vi "Dashboard Main.vi"() -> ()   [LabVIEW 2017]
uses:
  <vilib>/Utility/miscctls.llb/LVRowAndColumnTypeDef.ctl
  <vilib>/event_ctls.llb/eventvkey.ctl
  <vilib>/MakerHub/LINX/Public/Peripherals/Digital/Digital Write 1 Chan.vi
  <vilib>/MakerHub/LINX/Public/Peripherals/Digital/Digital Write N Chans.vi
  <vilib>/MakerHub/LINX/Private/Local IO/LinxDigitalWrite.vi
  <vilib>/MakerHub/LINX/Public/Utilities/Check Channel.vi
  <vilib>/Rock Robotics/Network Tables/NT Read Numeric Array.vi
  <vilib>/Rock Robotics/WPI/Dashboard/WPI_DashboardLogging Global.vi
  <vilib>/MakerHub/LINX/Public/Utilities/Open Serial.vi
  <vilib>/Rock Robotics/Network Tables/NT Read Boolean.vi
  <vilib>/MakerHub/LINX/Private/Utilties/Generate Error.vi
  <vilib>/MakerHub/LINX/LMH-LINX.lvlib
panel:
  in  "Camera Settings Right":T1={"Frame Rate"=30, "Compression"=30, "Size"=1, "DB Camera Config"=FALSE} {"Frame Rate" scale=1.0..30.0; "Compression" scale=100.0..-1.0; "Size" items=["640x480", "320x240", "160x120"]}
  in  "Camera Name Right":string(combo)="No Camera Selection"
  out "Camera Info":cluster{"Mbps LED":bool, "Mbps":dbl, "fps":dbl} {"fps" format="%#.1g"; "Mbps" format="%#.1g"}
  in  "Camera Settings":T1={"Frame Rate"=30, "Compression"=30, "Size"=1, "DB Camera Config"=FALSE} {"Frame Rate" scale=1.0..30.0; "Compression" scale=100.0..-1.0; "Size" items=["640x480", "320x240", "160x120"]}
  in  "TCP":refnum<k5>
  in  "Rec Mode":enum32{"Stop", "Record", "Playback"}(radio)
  out "Robot IP":string
  out "Image Message":string="Timeout in Camera Communications"
  in  "Dashboard Tab":T2(tab)
  in  "Select Auto":string(combo)="Select Autonomous ..."
  out "NT Connection":bool
  out "MotorChart R":cluster{"Numeric":dbl, "Numeric":dbl}(graph)
  out "MotorChart L":cluster{"Numeric":dbl, "Numeric":dbl}(graph)
  out "MotorSliders R":cluster{"MotorSlide1":dbl, "MotorSlide2":dbl} {"MotorSlide2" scale=-1.0..1.0 scale format="%#_2e"; "MotorSlide1" scale=-1.0..1.0 scale format="%#_2e"}
  out "MotorSliders L":cluster{"MotorSlide1":dbl, "MotorSlide2":dbl} {"MotorSlide2" scale=-1.0..1.0 scale format="%#_2e"; "MotorSlide1" scale=-1.0..1.0 scale format="%#_2e"}
  out "Gyro":dbl(knob) scale=0.0..360.0
  out "JS1 Z":dbl(slide) scale=-1.0..1.0 scale format="%#_2e"
  out "JS1 Graph":cluster{"X":dbl, "Y":dbl}[](graph)
  out "JS1 Buttons":T3
  out "JS2 Z":dbl(slide) scale=-1.0..1.0 scale format="%#_2e"
  out "JS2 Graph":cluster{"X":dbl, "Y":dbl}[](graph)
  out "JS2 Buttons":T3
  out "Mode":T4(ring)=enum."Auto Disabled"
  out "Camera Image Right":T5(plugin-control)
  in  "DB/String 9":string
  in  "DB/String 8":string
  in  "DB/String 7":string
  in  "DB/String 6":string
  in  "DB/String 5":string
  in  "DB/String 4":string
  in  "DB/String 3":string
  in  "DB/String 2":string
  in  "DB/String 1":string
  in  "DB/String 0":string
  in  "DB/Slider 0":dbl(slide) scale=0.0..5.0
  in  "DB/Slider 1":dbl(slide) scale=0.0..5.0
  in  "DB/Slider 2":dbl(slide) scale=0.0..5.0
  in  "DB/Slider 3":dbl(slide) scale=0.0..5.0
  out "DB/LED 3":bool
  out "DB/LED 2":bool
  out "DB/LED 1":bool
  out "DB/LED 0":bool
  in  "DB/Button 3":bool
  in  "DB/Button 2":bool
  in  "DB/Button 1":bool
  in  "DB/Button 0":bool caption="New Name"
  in  "Test Slider":dbl(slide) scale=0.0..100.0 scale format="%#_3g"
  in  "On/Off":bool caption="Solenoid"
  in  "Test Name":u16(ring) items=["Select the test to run..."]
  in  "Test Tree":string(tree)
  in  "Motor":cluster{"Value":dbl, "Enable":bool} {"Value" scale=-1.0..1.0 scale format="%#_3g"}
  out "Progress":T6 {"Test Progress" scale=0.0..100.0}
  in  "Rev/Fwd":cluster{"Forward":bool, "Reverse":bool}
  in  "Test Ring":u16(ring) items=["Monochrome", "Color"]
  out "Cmd Status":string
  in  "Execute Command":bool
  in  "Command Params":string[][](table)
  in  "Command Selection":i32(listbox)
  in  "CheckList":i32(listbox)
  out "Tree":string(tree)
  out "Camera Image":T5(plugin-control)
  out "Background":bool
  in  "Camera Name":string(combo)="No Camera Selection"
  # "HW"
  # "HW"
  # "Joysticks"
  # "Drive Motors"
  # "Front"
  # "Right"
  # "Left"
  # "Back"
  # "This tab is a great place for autonomous settings and robot-specific values.\nPlace controls and indicators inside this tab and match name to\nDashboard Variables on robot. You can also delete this comment."
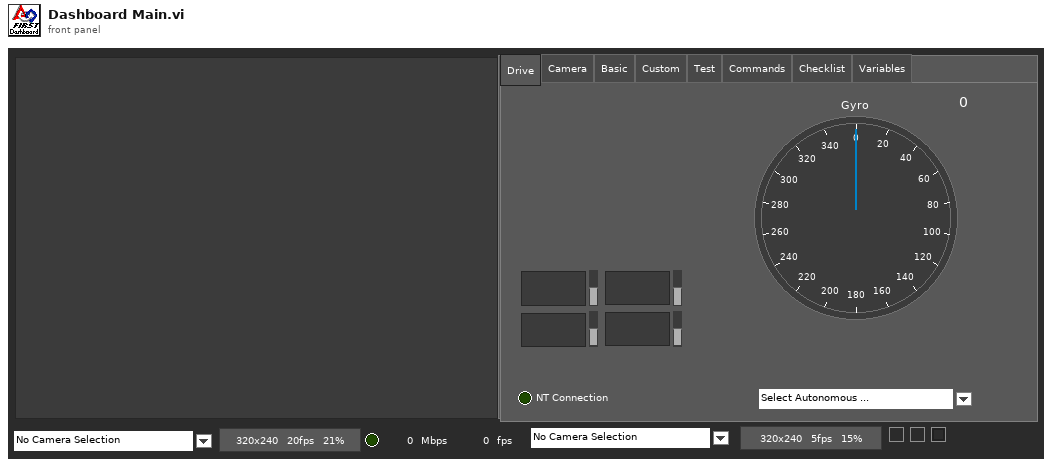
[diagram p1: front panel]
types:
  T1 = cluster{"Frame Rate":i32, "Compression":i32, "Size":u16, "DB Camera Config":bool}
  T2 = enum32{"Drive", "Camera", "Basic", "Custom", "Test", "Commands", "Checklist", "Variables"}
  T3 = cluster{bool, bool, bool, bool, bool, bool, bool, bool, bool, bool, bool, bool}
  T4 = enum8{"Tele-Op Disabled", "Tele-Op Enabled", "Auto Disabled", "Auto Enabled", "Test Disabled", "Test Enabled", "Disconnected", "No Code", "E-Stop"}
  T5 = typedef "IMAQ Image.ctl" = refnum<image>
  T6 = cluster{"Test Progress":u8, "Test Progress Text":string}
  T7 = cluster{"Save Path":path, "Interval (s)":dbl, "Keep":i32}
  T8 = typedef "Image Type" = u32
  T9 = cluster{"IDs":cluster{"RPC field ID":u16, "Unique ID":u16}, "String":string}
  T10 = typedef "LMH-LINX.lvlib/LINX Ref.ctl" = cluster{"IO":T11, "Interface":T12, "LINX Device Config":T13}
  T11 = typedef "LMH-LINX.lvlib/Platform.ctl" = enum16{"Remote", "Local"}
  T12 = typedef "LMH-LINX.lvlib/Interface.ctl" = enum16{"Serial", "TCP"}
  T13 = typedef "LMH-LINX.lvlib/Device.lvlib/LINX Device Config.ctl" = cluster{"Interface":T12, "COM Port":refnum<visa-resource-name>, "TCP Configuration":T14, "Device Family":u8, "Device ID":u8, "Device Name":string, "TCP Ref":refnum<k5>, "Channels":T15}
  T14 = typedef "LMH-LINX.lvlib/Device.lvlib/TCP Config.ctl" = cluster{"IP Address":string, "Port":u16}
  T15 = typedef "LMH-LINX.lvlib/Channels.ctl" = cluster{"DI":u8[], "DO":u8[], "AI":u8[], "AO":u8[], "PWM":u8[], "QE":u8[], "UART":u8[], "I2C 2":u8[], "SPI":u8[], "CAN":u8[], "Servo":u8[], "AI Ref (V)":dbl, "AI Resolution (Bits)":u8, "AO Ref (V)":dbl, "AO Resolution (Bits)":u8}
  T16 = cluster{"Error Strings":string, "Disable Counts":cluster{u16, u16}, "Rail Faults":cluster{u16, u16, u16}, "Robot IP":string, "DB Mode":u8, "Event Info":cluster{"Name":string, "Type":u8, "Number":u16, "Replay":u8}}
  T17 = cluster{"Storage":cluster{"Disk Free":u64, "RAM Block":u32, "RAM free":u32}, "CPU Utilization":cluster{"CPU % ISR":sgl, "CPU % Time Crit":sgl, "CPU % Timed Str":sgl, "CPU % High":sgl, "CPU % Above":sgl, "CPU % Normal":sgl, "CPU % Low":sgl}, "CAN":cluster{"% Bus Utilization":sgl, "Bus Off Cnt":u32, "TX_FIFO Full Cnt":u32, "Receive Error Cnt":u8, "Transmit Error Cnt":u8}, "HID":cluster{"HID Outputs":u32, "Rumble Low":u16, "Rumble High":u16}[]}
  T18 = cluster{"Status bits":cluster{"Test Mode":bool, "Autonomous":bool, "Enabled":bool, "Code Start":bool, "Brownout":bool, "Reserved 2":bool, "Reserved 3":bool, "E-Stop":bool}, "Code Trace":cluster{"Disabled":bool, "TeleOp":bool, "Auto":bool, "Test":bool}, "Controller Type":enum16{"unknown", "cRIO", "roboRio"}, "Code?":enum16{"unknown", "noCode", "code"}, "Battery V":dbl}
  T19 = cluster{"Control Bits":cluster{"TestMode":bool, "Autonomous":bool, "Enabled":bool, "FMS Present":bool, bool, bool, bool, "E-Stop":bool}, "Team Station ":u8, "Countdown":sgl, "Joystick Values":cluster{"Axes":dbl[], "Buttons":bool[], "POVs":i16[]}[]}
  T20 = cluster{"Axes":dbl[], "Buttons":bool[], "POVs":i16[]}[]
  T21 = cluster{"Axes":dbl[], "Buttons":bool[], "POVs":i16[]}
  T22 = cluster{"Buttons[0]":bool, "Buttons[1]":bool, "Buttons[2]":bool, "Buttons[3]":bool, "Buttons[4]":bool, "Buttons[5]":bool, "Buttons[6]":bool, "Buttons[7]":bool, "Buttons[8]":bool, "Buttons[9]":bool, "Buttons[10]":bool, "Buttons[11]":bool}
  T23 = cluster{"Camera Image":refnum<vi>, "Dashboard Tab":refnum<vi>, "Background":refnum<vi>, "Rec Mode":refnum<vi>, "Test Slider":refnum<vi>, "On/Off ":refnum<vi>, "Test Ring":refnum<vi>, "Rev/Fwd":refnum<vi>, "Test Name":refnum<vi>, "Motor":refnum<vi>, "Progress":refnum<vi>, "CheckList":refnum<vi>, "Tree":refnum<vi>, "Test Tree":refnum<vi>, "Command Params":refnum<vi>, "Command Selection":refnum<vi>, "Execute Command":refnum<vi>, "Cmd Status":refnum<vi>, "Camera Settings":refnum<vi>, "Camera Name":refnum<vi>, "Camera Info":refnum<vi>, "Camera Settings Right":refnum<vi>, "Camera Name Right":refnum<vi>, "Camera Image Right":refnum<vi>}
  T24 = cluster{"Camera Name":string, string, "Saved DB Images Info":cluster{"Save Path":path, "Interval (s)":dbl, "Keep":i32}}
  T25 = cluster{"Camera Name Right":string, string, "Saved DB Images Info":cluster{"Save Path":path, "Interval (s)":dbl, "Keep":i32}}
  T26 = cluster{"Operation":enum16{"Update", "Clear"}, "Color Box":u32}[]
  T27 = typedef "eventvkey.ctl" = enum16{"ASCII", "Enter", "Return", "Shift", "Ctrl", "Alt", "Cmd", "Opt", "Caps", "NumLock", "Clear", "Break", "Up", "Down", "Left", "Right", "Insert", "Delete", "Home", "End", "PageUp", "PageDown", "Escape", "Help", "Pause", "ScrollLock", "F1", "F2", "F3", "F4", "F5", "F6", "F7", "F8", "F9", "F10", "F11", "F12", "F13", "F14", "F15", "F16", "F17", "F18", "F19", "F20", "F21", "F22", "F23", "F24", "Play", "VolumeUp", "VolumeDown", "Mute", "Two Byte Char"}
  T28 = cluster{"Image Size":bool, "Image Type":bool, "Pixel Value":bool, "ROI Information":bool, "Zoom Factor":bool}
  T29 = cluster{"Operation":enum16{"Update", "Clear"}, "Color Box":u32}
  T30 = typedef "LVRowAndColumnTypeDef.ctl" = cluster{"Row":i32, "Column":i32}
  T31 = cluster{"Shift":bool, "Ctrl":bool, "Alt":bool, "Cmd":bool, "Opt":bool}
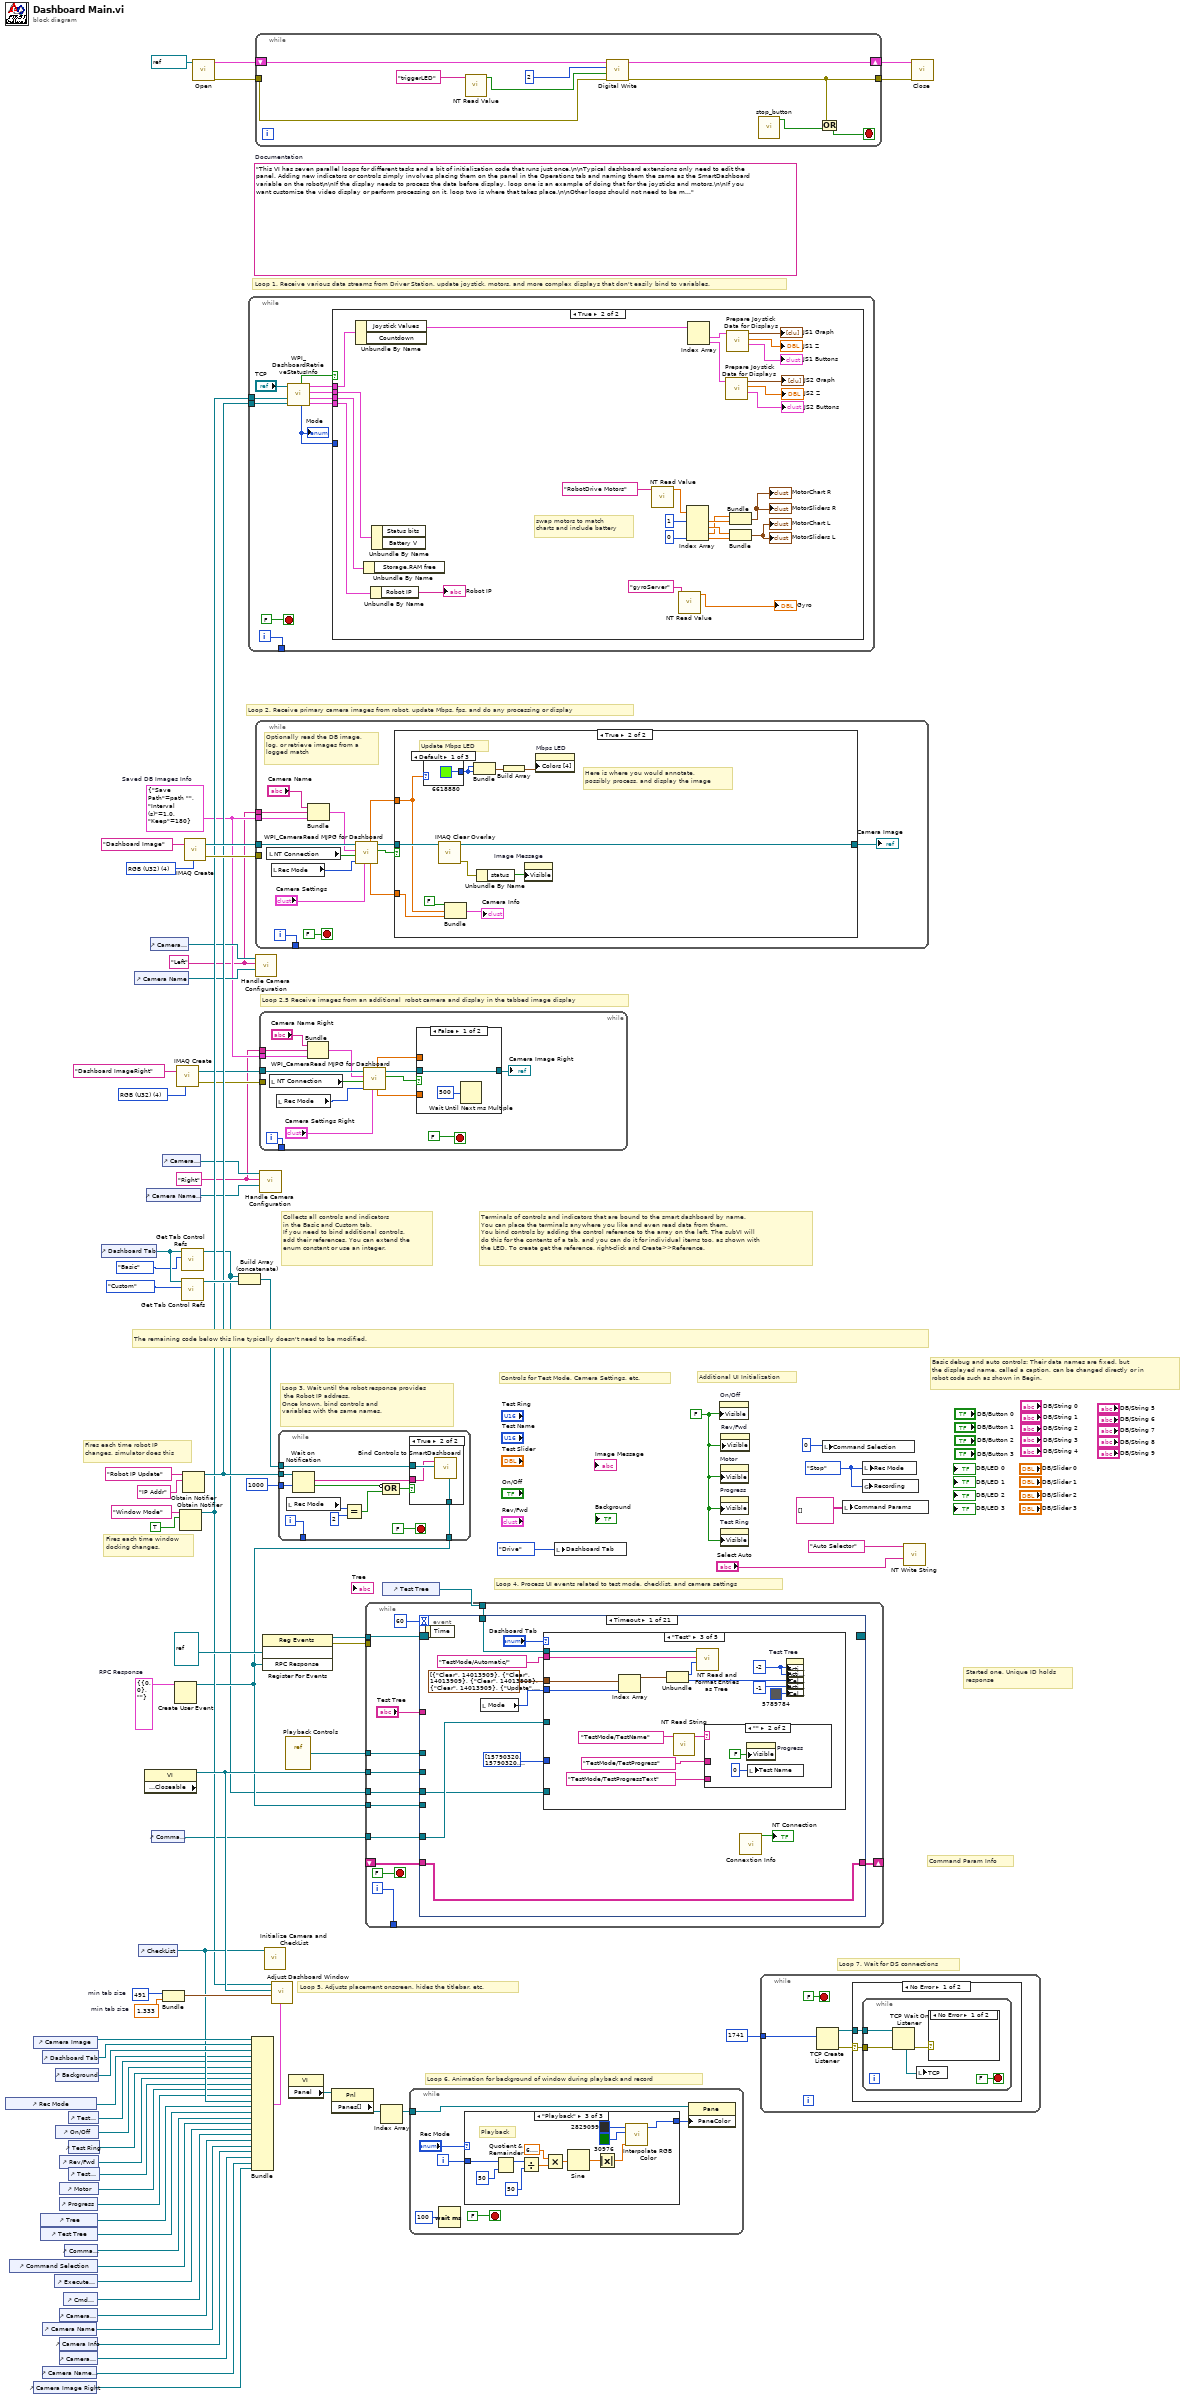
[diagram p0: block diagram]
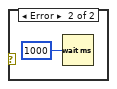
[diagram p3: hidden frame]
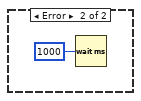
[diagram p4: hidden frame]
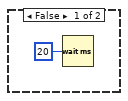
[diagram p5: hidden frame]
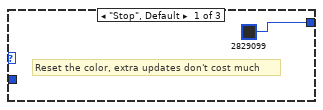
[diagram p6: hidden frame]
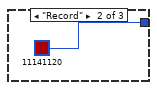
[diagram p7: hidden frame]
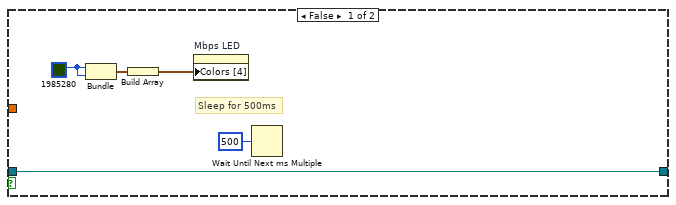
[diagram p9: hidden frame]
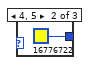
[diagram p10: hidden frame]
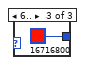
[diagram p11: hidden frame]
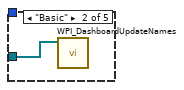
[diagram p13: hidden frame]
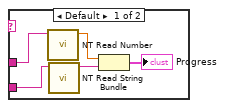
[diagram p14: hidden frame]
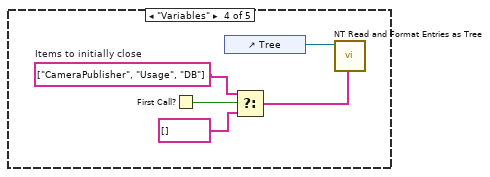
[diagram p15: hidden frame]
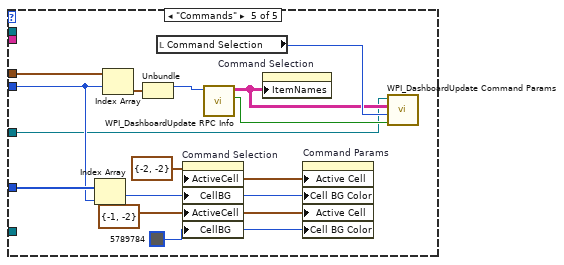
[diagram p16: hidden frame]
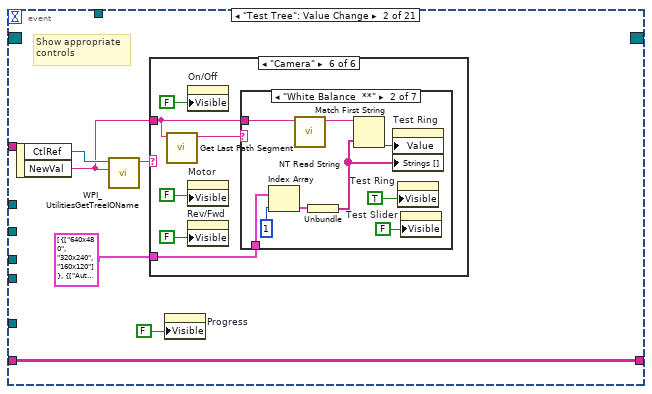
[diagram p17: hidden frame]
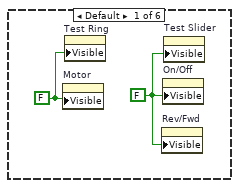
[diagram p18: hidden frame]
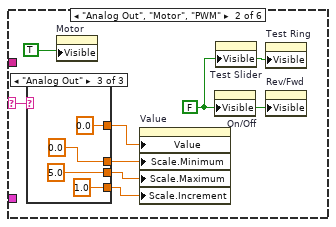
[diagram p19: hidden frame]
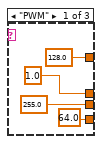
[diagram p20: hidden frame]
diagram:
  w8 = T7 {"Save Path"=path "", "Interval (s)"=1.0, "Keep"=180}  # Saved DB Images Info
  w7 = "Right"
  w6 = "Left"
  w18 = T8 4 items=["Grayscale (U8)", "Grayscale (I16)", "Grayscale (SGL)", "Complex (CSG)", "RGB (U32)", "HSL (U32)", "RGB (U64)"] ("Image Type")
  w34 = T9 {"IDs"={"RPC field ID"=0, "Unique ID"=0}, "String"=""}  # RPC Response
  w57 = 491  # min tab size
  w56 = 1.333  # min tab size
  w64 = enum32{"Stop", "Record", "Playback"}."Stop" ("Rec Mode")
  w41 = FALSE ("Visible")
  (unwired) "This VI has seven parallel loops for different tasks and a bit of initialization code that runs just once.\n\nTypical dashboard extensions only need to edit the panel. Adding new indicators or controls simply involves placing them on the panel in the Operations tab and naming them the same as the SmartDashboard variable on the robot\n\nIf the display needs to process the data before display, loop one is an example of doing that for the joysticks and motors.\n\nIf you want customize the video display or perform processing on it, loop two is where that takes place.\n\nOther loops should not need to be modified. They are pretty standard, and document the task they perform."  # Documentation
  w81 = T8 4 items=["Grayscale (U8)", "Grayscale (I16)", "Grayscale (SGL)", "Complex (CSG)", "RGB (U32)", "HSL (U32)", "RGB (U64)"] ("Image Type")
  # "Loop 2.5 Receive images from an additional  robot camera and display in the tabbed image display"
  # "Command Param Info"
  # "Started one, Unique ID holds\nresponse"
  # "Loop 7. Wait for DS connections"
  # "Basic debug and auto controls: Their data names are fixed, but\nthe displayed name, called a caption, can be changed directly or in\nrobot code such as shown in Begin."
  # "Controls for Test Mode, Camera Settings, etc."
  # "Additional UI Initialization"
  # "Loop 6. Animation for background of window during playback and record"
  # "Fires each time robot IP\nchanges, simulator does this"
  # "Fires each time window\ndocking changes."
  # "Collects all controls and indicators\nin the Basic and Custom tab.\nIf you need to bind additional controls,\nadd their references. You can extend the\nenum constant or use an integer."
  # "The remaining code below this line typically doesn't need to be modified."
  # "Loop 4. Process UI events related to test mode, checklist, and camera settings"
  # "Terminals of controls and indicators that are bound to the smart dashboard by name.\nYou can place the terminals anywhere you like and even read data from them.\nYou bind controls by adding the control reference to the array on the left. The subVI will\ndo this for the contents of a tab, and you can do it for individual items too, as shown with\nthe LED. To create get the reference, right-click and Create>>Reference."
  # "Loop 3. Wait until the robot response provides\n the Robot IP address.\nOnce known, bind controls and\nvariables with the same names."
  # "Loop 5. Adjusts placement onscreen, hides the titlebar, etc."
  # "Loop 1. Receive various data streams from Driver Station, update joystick, motors, and more complex displays that don't easily bind to variables."
  # "Loop 2. Receive primary camera images from robot, update Mbps, fps, and do any processing or display"
  n1 = control-ref of="Rec Mode"() -> (w47:refnum<vi>)
  n2 = control-ref of="Command Selection"() -> (w33:refnum<vi>)
  n3 = control-ref of="Camera Image Right"() -> (w11:refnum<vi>)
  n4 = control-ref of="Camera Image"() -> (w59:refnum<vi>)
  n5 = control-ref of="Tree"() -> (w51:refnum<vi>)
  n6 = control-ref of="Test Tree"() -> (w50:refnum<vi>)
  n7 = control-ref of="Dashboard Tab"() -> (w58:refnum<vi>)
  n8 = control-ref of="Camera Name"() -> (w24:refnum<vi>)
  n9 = control-ref of="Camera Name Right"() -> (w12:refnum<vi>)
  n10 = control-ref of="Execute Command"() -> (w35:refnum<vi>)
  n11 = control-ref of="Background"() -> (w54:refnum<vi>)
  n12 = control-ref of="On/Off"() -> (w45:refnum<vi>)
  n13 = control-ref of="Progress"() -> (w42:refnum<vi>)
  n14 = control-ref of="Camera Settings"() -> (w25:refnum<vi>)
  n15 = control-ref of="Camera Info"() -> (w23:refnum<vi>)
  n16 = control-ref of="Camera Settings Right"() -> (w13:refnum<vi>)
  n17 = control-ref of="Rev/Fwd"() -> (w43:refnum<vi>)
  n18 = control-ref of="Motor"() -> (w48:refnum<vi>)
  n19 = control-ref of="Cmd Status"() -> (w29:refnum<vi>)
  n20 = control-ref of="Command Params"() -> (w36:refnum<vi>)
  n21 = control-ref of="Test Slider"() -> (w46:refnum<vi>)
  n22 = control-ref of="Test Ring"() -> (w44:refnum<vi>)
  n23 = control-ref of="Test Name"() -> (w49:refnum<vi>)
  n24 = control-ref of="Dashboard Tab"() -> (w62:refnum<vi>)
  n25 = control-ref of="Camera Name"() -> (w26:refnum<vi>)
  n26 = control-ref of="CheckList"() -> (w52:refnum<vi>)
  n27 = property class="VI" props=["Front Panel.Closeable"]() -> (reference out=w63:refnum<vi>)  [unwired: 2 in, 2 out]
  n28 = control-ref of="Camera Name Right"() -> (w14:refnum<vi>)
  n29 = control-ref of="Camera Settings"() -> (w27:refnum<vi>)
  n30 = control-ref of="Command Params"() -> (w28:refnum<vi>)
  n31 = control-ref of="Camera Settings Right"() -> (w15:refnum<vi>)
  n32 = Bundle("min tab size"=w57, "min tab size"=w56) -> (w55:cluster{"min tab size":i32, "min tab size":dbl})  [unwired: 1 in]
  n33 = Create User Event(user event datatype=w34) -> (user event=w30:refnum<user-event>)  [unwired: 1 in, 1 out]
  n34 = call "IMAQ Create"("Image Name"="Dashboard ImageRight", "Image Type"=w18) -> ("New Image"=w17:T5, "error out"=w16:errorcluster)  [unwired: 2 in, 1 out]
  n35 = Obtain Notifier(name (unnamed)="Window Mode", notification data type=TRUE) -> (notifier out=w39:refnum<notifier>)  [unwired: 2 in, 2 out]
  n36 = call <vilib>:"Get Tab Control Refs.vi"("Page Index"=T2."Basic" ("Dashboard Tab"), "TabControl in"=w62) -> ("ControlsOnPage"=w22:refnum<vi>[])  [unwired: 9 in]
  n37 = call <vilib>:"Get Tab Control Refs.vi"("Page Index"=T2."Custom" ("Dashboard Tab"), "TabControl in"=w62) -> ("ControlsOnPage"=w61:refnum<vi>[])  [unwired: 9 in]
  n38 = Obtain Notifier(name (unnamed)="Robot IP Update", notification data type="IP Addr" ("name (unnamed)")) -> (notifier out=w40:refnum<notifier>)  [unwired: 2 in, 2 out]
  n39 = call "IMAQ Create"("Image Name"="Dashboard Image", "Image Type"=w81) -> ("New Image"=w79:T5, "error out"=w78:errorcluster)  [unwired: 2 in, 1 out]
  n40 = call-poly <vilib>:"Open.vi"("Serial Port"=refnum<visa-resource-name> "N/A") -> ("Error Out"=w3:errorcluster, "LINX Resource"=w4:T10)  [unwired: 8 in, 1 out]
  n41 = Build Array (concatenate)(w22, w61) -> (w60:refnum<vi>[])
  n42 = while {
    tunnel: [w91] -> _
    tunnel: w40 -> [w85]
    tunnel: w39 -> [w82]
    i -> [w91]
    stop <- FALSE stop-if-true
    n43 = call <vilib>:"WPI_DashboardRetrieveStatusInfo.vi"("Binding Refnum"=w85, "Window Mode Notifier"=w82, "TCP Cnx"="TCP") -> ("Power and Errors"=w86:T16, "Robot Metrics"=w89:T17, "Status Info"=w90:T18, "Control Info"=w87:T19, "Robot Mode"=w84:T4, "Process?"=w88:bool)  [unwired: 3 in]
    "Mode" <- w84
    n44 = case shown="True" w88 {
      tunnel: w90 -> [_ w119]
      tunnel: w89 -> [_ w118]
      tunnel: w87 -> [_ w117]
      tunnel: w86 -> [_ w116]
      tunnel: w84 -> [_ _]
      frame False {
        n45 = Wait (ms)(milliseconds to wait=u32 20) -> ()  [unwired: 1 out]
      }
      frame True {
        # "swap motors to match\ncharts and include battery"
        n46 = Unbundle By Name(w117) -> ("Joystick Values"=w107:T20)  [unwired: 1 out]
        n47 = Unbundle By Name(w118) -> ()  [unwired: 1 out]
        n48 = Unbundle By Name(w116) -> ("Robot IP"=→"Robot IP":string)
        n49 = Unbundle By Name(w119) -> ()  [unwired: 2 out]
        n50 = call-poly <vilib>:"NT Read Value.vi"("Name"="RobotDrive Motors") -> ("Numeric Array"=w97:dbl[])  [unwired: 9 in, 1 out]
        n51 = call-poly <vilib>:"NT Read Value.vi"("Name"="gyroServer") -> ("Numeric"=→"Gyro":dbl)  [unwired: 9 in, 1 out]
        n52 = Index Array(array=w97, index #1=1, index #4=0) -> (element #1=w111:dbl, element #2=w112:dbl, element #3=w110:dbl, element #4=w115:dbl)  [unwired: 2 in]
        n53 = Index Array(array=w107) -> (element #1=w106:T21, element #2=w102:T21)  [unwired: 2 in]
        n54 = call "Prepare Joystick Data for Displays.vi"("Joystick Values"=w102) -> ("Buttons"=→"JS2 Buttons":T22, "Z Axis"=→"JS2 Z":dbl, "Cartesian Data"=→"JS2 Graph":cluster{"X axis":dbl, "X axis":dbl}[])  [unwired: 8 in]
        n55 = call "Prepare Joystick Data for Displays.vi"("Joystick Values"=w106) -> ("Buttons"=→"JS1 Buttons":T22, "Z Axis"=→"JS1 Z":dbl, "Cartesian Data"=→"JS1 Graph":cluster{"X axis":dbl, "X axis":dbl}[])  [unwired: 8 in]
        n56 = Bundle("Numeric"=w110, "Numeric"=w111) -> (→"MotorChart R" →"MotorSliders R":cluster{"Numeric":dbl, "Numeric":dbl})  [unwired: 1 in]
        n57 = Bundle("Numeric"=w112, "Numeric"=w115) -> (→"MotorChart L" →"MotorSliders L":cluster{"Numeric":dbl, "Numeric":dbl})  [unwired: 1 in]
      }
    }
  }
  n58 = Bundle("Camera Image"=w59, "Dashboard Tab"=w58, "Background"=w54, "Rec Mode"=w47, "Test Slider"=w46, "On/Off"=w45, "Test Ring"=w44, "Rev/Fwd"=w43, "Test Name"=w49, "Motor"=w48, "Progress"=w42, "CheckList"=w52, "Tree"=w51, "Test Tree"=w50, "Command Params"=w36, "Command Selection"=w33, "Execute Command"=w35, "Cmd Status"=w29, "Camera Settings"=w25, "Camera Name"=w24, "Camera Info"=w23, "Camera Settings Right"=w13, "Camera Name Right"=w12, "Camera Image Right"=w11) -> (w53:T23)  [unwired: 1 in]
  n59 = call "Handle Camera Configuration.vi"("CameraNameRef"=w26, "Display Name"=w6, "ClusterRef"=w27) -> ()  [unwired: 9 in]
  n60 = while {
    shift-right: [w127] -> w2
    shift-left: w4 -> [w128]
    tunnel: w3 -> [w125]
    tunnel: [w126] -> w1
    stop <- w123 stop-if-true
    n61 = call-poly <vilib>:"NT Read Value.vi"("Name"="triggerLED") -> ("Boolean"=w120:bool)  [unwired: 9 in, 1 out]
    n62 = call-poly <vilib>:"Digital Write.vi"("Error In"=w125, "Output Value"=w120, "DO Channel"=u8 2 ("AO Channel"), "LINX Resource"=w128) -> ("Error Out"=w126:errorcluster, "LINX Resource"=w127:T10)  [unwired: 6 in]
    n63 = call "stop_button.vi"() -> ("Boolean"=w122:bool)  [unwired: 11 in]
    n64 = Or(x=w126, y=w122) -> (x .or. y?=w123:bool)
  }
  n65 = while {
    tunnel: w79 -> [w141]
    tunnel: w78 -> [_]
    tunnel: [w142] -> _
    tunnel: w8 -> [w132]
    tunnel: w6 -> [w129]
    i -> [w142]
    stop <- FALSE stop-if-true
    # "Optionally read the DB image,\nlog, or retrieve images from a\nlogged match"
    n66 = local read "NT Connection"() -> (w133:bool)
    n67 = local read "Rec Mode"() -> (w137:enum32{"Stop", "Record", "Playback"})
    n68 = Bundle("Camera Name"="Camera Name", w129, "Saved DB Images Info"=w132) -> (w131:T24)  [unwired: 1 in]
    n69 = call <vilib>:"WPI_CameraRead MJPG for Dashboard.vi"("Camera Settings"="Camera Settings", "Rec Mode"=w137, "NT Connection"=w133, "Capture Info"=w131, "Refnum in"=w141) -> ("Active"=w139:bool, "Refnum out"=w140:T5, "FPS"=w138:dbl, "Bandwidth (Mbps)"=w136:dbl)  [unwired: 3 in]
    n70 = case shown="True" w139 {
      tunnel: w140 -> [w144 w155]
      tunnel: w136 -> [_ w152]
      tunnel: w138 -> [_ w153]
      tunnel: [w144 w149] -> w134
      frame False {
        w146 = u32 1985280 ("Color Box")
        # "Sleep for 500ms"
        n71 = Bundle("Color Box"=w146, "Color Box"=w146) -> (w147:cluster{"Color Box":u32, "Color Box":u32})  [unwired: 1 out]
        n72 = Build Array(w147) -> (w145:cluster{"Color Box":u32, "Color Box":u32}[])
        n73 = property on="Mbps LED" class="Bool (strict)"("Colors [4]"=w145) -> ()  [unwired: 2 in, 2 out]
        n74 = Wait Until Next ms Multiple(millisecond multiple=u32 500) -> ()  [unwired: 1 out]
      }
      frame True {
        # "Here is where you would annotate,\npossibly process, and display the image"
        # "Update Mbps LED"
        n75 = case shown="Default" w152 {
          tunnel: [u32 6618880 ("Color Box") u32 16776722 ("Color Box") u32 16716800 ("Color Box")] -> w156
          frame Default {
          }
          frame 4, 5 {
          }
          frame 6.. {
          }
        }
        n76 = call "IMAQ Clear Overlay"("Image"=w155) -> ("error out"=w158:errorcluster, "Image Out"=w149:T5)  [unwired: 2 in, 7 out]
        n77 = Bundle(FALSE, "Bandwidth (Mbps)"=w152, "FPS"=w153) -> (→"Camera Info":cluster{bool, "Bandwidth (Mbps)":dbl, "FPS":dbl})  [unwired: 1 in]
        n78 = Bundle("Color Box"=w156, "Color Box"=w156) -> (w157:cluster{"Color Box":u32, "Color Box":u32})  [unwired: 1 out]
        n79 = Unbundle By Name(w158) -> ("status"=w159:bool)
        n80 = Build Array(w157) -> (w154:cluster{"Color Box":u32, "Color Box":u32}[])
        n81 = property on="Image Message" class="Str"("Visible"=w159) -> ()  [unwired: 2 in, 2 out]
        n82 = property on="Mbps LED" class="Bool (strict)"("Colors [4]"=w154) -> ()  [unwired: 2 in, 2 out]
      }
    }
    "Camera Image" <- w134
  }
  n83 = call "Handle Camera Configuration.vi"("CameraNameRef"=w14, "Display Name"=w7, "ClusterRef"=w15) -> ()  [unwired: 9 in]
  n84 = while {
    tunnel: w17 -> [w177]
    tunnel: w16 -> [_]
    tunnel: [w172] -> _
    tunnel: w8 -> [w166]
    tunnel: w7 -> [w163]
    i -> [w172]
    stop <- FALSE stop-if-true
    n85 = local read "NT Connection"() -> (w167:bool)
    n86 = local read "Rec Mode"() -> (w176:enum32{"Stop", "Record", "Playback"})
    n87 = Bundle("Camera Name Right"="Camera Name Right", w163, "Saved DB Images Info"=w166) -> (w165:T25)  [unwired: 1 in]
    n88 = call <vilib>:"WPI_CameraRead MJPG for Dashboard.vi"("Camera Settings"="Camera Settings Right", "Rec Mode"=w176, "NT Connection"=w167, "Capture Info"=w165, "Refnum in"=w177) -> ("Active"=w171:bool, "Refnum out"=w174:T5, "FPS"=w169:dbl, "Bandwidth (Mbps)"=w170:dbl)  [unwired: 3 in]
    n89 = case shown="False" w171 {
      tunnel: w174 -> [w178 w180]
      tunnel: w170 -> [_ _]
      tunnel: w169 -> [_ _]
      tunnel: [w178 w180] -> w168
      frame False {
        n90 = Wait Until Next ms Multiple(millisecond multiple=u32 500) -> ()  [unwired: 1 out]
      }
      frame True {
      }
    }
    "Camera Image Right" <- w168
  }
  n91 = register-events(refnum<vi> refnum, w30) -> (reference out=w68:refnum<event-registration>, error out=w67:errorcluster)  [unwired: 2 in]
  n92 = call "Initialize Camera and CheckList.vi"("ListBox in"=w52) -> ()  [unwired: 11 in]
  n93 = call "Adjust Dashboard Window.vi"("Sizing Refnums"=w53, "Size Constraints"=w55, "VI"=w63, "WIn Mode"=w39) -> ()  [unwired: 8 in]
  n94 = while {
    tunnel: w60 -> [w192]
    tunnel: w40 -> [w190]
    tunnel: [w188] -> _
    tunnel: u32 1000 ("milliseconds to wait") -> [w187]
    tunnel: w30 -> [w181]
    i -> [w188]
    stop <- FALSE stop-if-true
    n95 = local read "Rec Mode"() -> (w183:enum32{"Stop", "Record", "Playback"})
    n96 = Wait on Notification(notifier=w190, timeout in ms (-1)=w187) -> (notification=w189:string, timed out?=w185:bool)  [unwired: 2 in, 2 out]
    n97 = Equal?(x=w183, y=u16 2 ("Rec Mode")) -> (x = y?=w184:bool)
    n98 = Compound Arithmetic op=OR(invert w185, w184) -> (w186:bool)
    n99 = case shown="True" w186 {
      tunnel: w192 -> [_ w195]
      tunnel: w189 -> [_ w194]
      tunnel: w181 -> [_ w193]
      frame False {
      }
      frame True {
        n100 = call <vilib>:"Bind Controls to SmartDashboard.vi"("RPC ref"=w193, "Bound Control Refs"=w195, "Server IP Address"=w194) -> ()  [unwired: 9 in]
      }
    }
  }
  n101 = vi-ref "Playback Controls.vi"() -> (w69:refnum<vi>)
  n102 = property class="VI"() -> ("Panel"=w71:refnum<vi>)  [unwired: 2 in, 2 out]
  n103 = property class="Pnl"(reference=w71) -> ("Panes[]"=w72:refnum<vi>[])  [unwired: 1 in, 2 out]
  n104 = Index Array(array=w72) -> (element=w70:refnum<vi>)  [unwired: 1 in]
  n105 = control-ref of="Test Tree"() -> (w73:refnum<vi>)
  n106 = while {
    tunnel: [w205] -> _
    tunnel: w73 -> [w204]
    tunnel: w69 -> [w203]
    tunnel: w68 -> [w202]
    tunnel: w67 -> [_]
    tunnel: w63 -> [w201]
    tunnel: w30 -> [w200]
    tunnel: w28 -> [w199]
    shift-right: [w198] -> _
    shift-left: _ -> [w197]
    tunnel: w22 -> [w196]
    i -> [w205]
    stop <- FALSE stop-if-true
    n107 = event shown="[0] Timeout" {
      selector: w202 -> [_ _ _ _ _ _ _ _ _ _ _ _ _ _ _ _ _ _ _ _ _]
      dyn-events: [_ _ _ _ _ _ _ _ _ _ _ _ _ _ _ _ w465 _ _ _ _] -> _
      timeout: u32 60 ("milliseconds to wait") -> [_ _ _ _ _ _ _ _ _ _ _ _ _ _ _ _ _ _ _ _ _]
      tunnel: w204 -> [w217 _ _ _ _ _ _ _ _ _ _ _ _ _ _ _ _ _ _ _ _]
      tunnel: "Test Tree" -> [_ _ _ _ _ _ _ _ _ _ _ w432 w440 w442 w446 w454 _ _ _ _ _]
      tunnel: w203 -> [_ _ _ _ _ _ _ _ _ _ _ _ _ _ _ _ w467 _ w485 _ _]
      tunnel: w201 -> [_ _ _ _ _ _ _ _ _ _ _ _ _ _ _ _ w463 _ _ _ _]
      tunnel: w200 -> [_ _ _ _ _ _ _ _ _ _ _ _ _ _ _ _ w461 _ _ _ _]
      tunnel: w199 -> [w212 _ _ _ _ _ w383 _ _ _ _ _ _ _ _ _ _ _ _ _ _]
      tunnel: [w211 w260 w362 w367 w376 w380 w381 w390 w400 w407 w419 w431 w438 w441 w445 w453 w460 w480 w482 w486 w499] -> w198
      tunnel: w197 -> [w211 w260 w362 w367 w376 w380 w381 _ _ w407 w419 w431 w438 w441 w445 w453 w460 w480 w482 w486 w499]
      tunnel: w196 -> [w209 _ _ _ _ _ _ _ _ _ _ _ _ _ _ _ _ _ _ _ _]
      event Timeout {
        n108 = event-data() -> ()  [unwired: 1 in, 1 out]
        n109 = local read "Mode"() -> (w214:T4)
        n110 = case shown="\"Test\"" "Dashboard Tab" {
          tunnel: w217 -> [_ _ w233 _ _]
          tunnel: "TestMode/Automatic/" ("Name Pattern") -> [_ _ w232 _ _]
          tunnel: T26 [{"Operation"=enum."Clear", "Color Box"=14013909}, {"Operation"=enum."Clear", "Color Box"=14013909}, {"Operation"=enum."Clear", "Color Box"=14013909}, {"Operation"=enum."Clear", "Color Box"=14013909}, {"Operation"=enum."Update", "Color Box"=14013909}, {"Operation"=enum."Update", "Color Box"=16777215}, {"Operation"=enum."Clear", "Color Box"=14013909}, {"Operation"=enum."Clear", "Color Box"=14013909}, {"Operation"=enum."Clear", "Color Box"=14013909}] -> [_ _ w225 _ w253]
          tunnel: w214 -> [_ _ w224 _ w252]
          tunnel: u32[] [15790320, 15790320, 15790320, 15790320, 16777215, 16777215, 15790320, 15790320, 15790320] -> [_ _ _ _ w258]
          tunnel: w212 -> [_ _ _ _ w246]
          tunnel: w209 -> [_ w219 _ _ _]
          frame "Custom", Default {
          }
          frame "Basic" {
            n111 = call <vilib>:"WPI_DashboardUpdateNames.vi"("Controls on Tab"=w219) -> ()  [unwired: 11 in]
          }
          frame "Test" {
            w231 = -2 ("Active Item:Row Number")
            n112 = Index Array(array=w225, index=w224) -> (element=w226:T29)
            n113 = Unbundle(w226) -> ("Operation"=w227:enum16{"Update", "Clear"}, "Color Box"=w228:u32)
            n114 = call <vilib>:"NT Read String.vi"("Name"="TestMode/TestName") -> ("String"=w222:string)  [unwired: 9 in, 1 out]
            n115 = call <vilib>:"NT Read and Format Entries as Tree.vi"("Operation"=w227, "Name Pattern"=w232, "Tree Refnum"=w233) -> ()  [unwired: 7 in, 2 out]
            n116 = case shown="\"\"" w222 {
              tunnel: "TestMode/TestProgress" ("Name") -> [w235 _]
              tunnel: "TestMode/TestProgressText" ("Name") -> [w234 _]
              frame Default {
                n117 = call <vilib>:"NT Read Number.vi"("Name"=w235) -> ("Numeric"=w236:dbl)  [unwired: 9 in, 1 out]
                n118 = call <vilib>:"NT Read String.vi"("Name"=w234) -> ("String"=w237:string)  [unwired: 9 in, 1 out]
                n119 = Bundle("Numeric"=w236, "String"=w237) -> (→"Progress":cluster{"Numeric":dbl, "String":string})  [unwired: 1 in]
              }
              frame "" {
                n120 = property on="Progress" class="Clust (strict)"("Visible"=FALSE) -> ()  [unwired: 2 in, 2 out]
                n121 = local write "Test Name"(u16 0) -> ()
              }
            }
            n122 = property on="Test Tree" class="Tree (strict)"("Active Item Row Number"=w231, "ActiveColNum"=w231, "CellBG"=w228, "Active Item Row Number"=-1 ("Active Item:Row Number"), "CellBG"=u32 5789784 ("Color Box")) -> ()  [unwired: 2 in, 2 out]
          }
          frame "Variables" {
            w243 = string[] ["CameraPublisher", "Usage", "DB"]  # Items to initially close
            n123 = First Call?() -> (First Call?: T/F=w244:bool)
            n124 = control-ref of="Tree"() -> (w245:refnum<vi>)
            n125 = Select(t=w243, s=w244, f=string[] []) -> (s? t:f=w241:string[])
            n126 = call <vilib>:"NT Read and Format Entries as Tree.vi"("Tags to  Close"=w241, "Tree Refnum"=w245) -> ()  [unwired: 8 in, 2 out]
          }
          frame "Commands" {
            w254 = u32 5789784 ("Color Box")
            w255 = T30 {"Row"=-1, "Column"=-2} ("Active Cell:Active Cell")
            w257 = T30 {"Row"=-2, "Column"=-2} ("Active Cell:Active Cell")
            n127 = Index Array(array=w258, index=w252) -> (element=w256:u32)
            n128 = Index Array(array=w253, index=w252) -> (element=w251:T29)
            n129 = Unbundle(w251) -> ("Operation"=w250:enum16{"Update", "Clear"})  [unwired: 1 out]
            n130 = local read "Command Selection"() -> (w249:i32)
            n131 = property on="Command Selection" class="MCListbox (strict)"("ActiveCell"=w257, "CellBG"=w256, "ActiveCell"=w255, "CellBG"=w254) -> ()  [unwired: 2 in, 2 out]
            n132 = call <vilib>:"WPI_DashboardUpdate RPC Info.vi"("Operation"=w250) -> ("update"=w248:bool, "commands"=w247:string[][])  [unwired: 9 in]
            n133 = property on="Command Selection" class="MCListbox (strict)"("ItemNames"=w247) -> ()  [unwired: 2 in, 2 out]
            n134 = property on="Command Params" class="Tbl (strict)"("Active Cell"=w257, "Cell BG Color"=w256, "Active Cell"=w255, "Cell BG Color"=w254) -> ()  [unwired: 2 in, 2 out]
            n135 = call <vilib>:"WPI_DashboardUpdate Command Params.vi"("Update"=w248, "NewVal"=w249, "Commands"=w247, "Param Tbl"=w246) -> ()  [unwired: 7 in, 1 out]
          }
        }
        n136 = call <vilib>:"Connextion Info.vi"() -> ("Connected"=→"NT Connection":bool)  [unwired: 10 in, 1 out]
      }
      event "Test Tree": Value Change {
        # "Show appropriate\ncontrols"
        n137 = event-data() -> ("CtlRef"=w263:refnum<vi>, "NewVal"=w261:string)  [unwired: 1 in]
        n138 = call <vilib>:"WPI_UtilitiesGetTreeIOName.vi"("NewVal"=w261, "TreeControl in"=w263) -> ("I/O Name"=w264:string)  [unwired: 9 in]
        n139 = case shown="\"Camera\"" w264 {
          selector: w264 -> [_ w271 _ w293 w302 _]
          tunnel: w261 -> [_ _ w290 w292 _ w309]
          tunnel: cluster{string[]}[] [{["640x480", "320x240", "160x120"]}, {["Auto", "Fixed indoor", "Fixed outdoor 1", "Fixed outdoor 2", "Fixed fluorescent 1", "Fixed fluorescent 2", "Hold current"]}, {["Auto", "Flicker-free 50 Hz", "Flicker-free 60 Hz", "Hold current"]}, {["None", "Prioritize frame rate", "Prioritize image quality"]}, {["Monochrome", "Color"]}] -> [_ _ _ _ _ w308]
          frame Default {
            w266 = FALSE ("Visible")
            w265 = FALSE ("Visible")
            n140 = property on="Motor" class="Clust (strict)"("Visible"=w265) -> ()  [unwired: 2 in, 2 out]
            n141 = property on="Test Ring" class="Ring (strict)"("Visible"=w265) -> ()  [unwired: 2 in, 2 out]
            n142 = property on="Rev/Fwd" class="Clust (strict)"("Visible"=w266) -> ()  [unwired: 2 in, 2 out]
            n143 = property on="On/Off" class="Bool (strict)"("Visible"=w266) -> ()  [unwired: 2 in, 2 out]
            n144 = property on="Test Slider" class="Slide (strict)"("Visible"=w266) -> ()  [unwired: 2 in, 2 out]
          }
          frame "Analog Out", "Motor", "PWM" {
            w272 = FALSE ("Visible")
            n145 = case shown="\"Analog Out\"" w271 {
              tunnel: [1.0 ("Value") -1.0 ("Value") 0.0 ("Value")] -> w270
              tunnel: [255.0 ("Value") 1.0 ("Value") 5.0 ("Value")] -> w269
              tunnel: [128.0 ("Value") 0.0 ("Value") 0.0 ("Value")] -> w268
              tunnel: [64.0 ("Value") 0.5 ("Value") 1.0 ("Value")] -> w267
              frame "PWM" {
              }
              frame "Motor", Default {
              }
              frame "Analog Out" {
              }
            }
            n146 = property on="Motor" class="Clust (strict)"("Visible"=TRUE) -> ()  [unwired: 2 in, 2 out]
            n147 = property on="Value" class="Slide (strict)"("Value"=w268, "Scale.Minimum"=w270, "Scale.Maximum"=w269, "Scale.Increment"=w267) -> ()  [unwired: 2 in, 2 out]
            n148 = property on="On/Off" class="Bool (strict)"("Visible"=w272) -> ()  [unwired: 2 in, 2 out]
            n149 = property on="Test Slider" class="Slide (strict)"("Visible"=w272) -> ()  [unwired: 2 in, 2 out]
            n150 = property on="Test Ring" class="Ring (strict)"("Visible"=w272) -> ()  [unwired: 2 in, 2 out]
            n151 = property on="Rev/Fwd" class="Clust (strict)"("Visible"=w272) -> ()  [unwired: 2 in, 2 out]
          }
          frame "Servo" {
            w288 = FALSE ("Visible")
            n152 = call <vilib>:"NT Read Number.vi"("Name"=w290) -> ("Numeric"=w289:dbl)  [unwired: 9 in, 1 out]
            n153 = property on="Test Slider" class="Slide (strict)"("Visible"=TRUE, "Scale.Maximum"=170.0 ("Scale.Range:Maximum")) -> ()  [unwired: 2 in, 2 out]
            n154 = local write "Test Slider"(w289) -> ()
            n155 = property on="Motor" class="Clust (strict)"("Visible"=w288) -> ()  [unwired: 2 in, 2 out]
            n156 = property on="Rev/Fwd" class="Clust (strict)"("Visible"=w288) -> ()  [unwired: 2 in, 2 out]
            n157 = property on="On/Off" class="Bool (strict)"("Visible"=w288) -> ()  [unwired: 2 in, 2 out]
            n158 = property on="Test Ring" class="Ring (strict)"("Visible"=w288) -> ()  [unwired: 2 in, 2 out]
          }
          frame "Relay", "Solenoid" {
            w291 = FALSE ("Visible")
            n159 = property on="Motor" class="Clust (strict)"("Visible"=w291) -> ()  [unwired: 2 in, 2 out]
            n160 = property on="Test Slider" class="Slide (strict)"("Visible"=w291) -> ()  [unwired: 2 in, 2 out]
            n161 = Search and Replace String(input string=w292, search string="/Value  **", replace string="/Direction") -> (result string=w298:string)  [unwired: 5 in, 3 out]
            n162 = property on="Test Ring" class="Ring (strict)"("Visible"=w291) -> ()  [unwired: 2 in, 2 out]
            n163 = call <vilib>:"NT Read String.vi"("Name"=w298) -> ("String"=w296:string)  [unwired: 9 in, 1 out]
            n164 = Equal?(x="Both directions", y=w296) -> (x = y?=w294:bool)
            n165 = Not(x=w294) -> (.not. x?=w295:bool)
            n166 = property on="Rev/Fwd" class="Clust (strict)"("Visible"=w294) -> ()  [unwired: 2 in, 2 out]
            n167 = property on="On/Off" class="Bool (strict)"("Visible"=w295, "Caption.Text"=w293) -> ()  [unwired: 2 in, 2 out]
          }
          frame "Compressor", "Digital Out" {
            w301 = FALSE ("Visible")
            # "Get direction and finish"
            n168 = property on="Motor" class="Clust (strict)"("Visible"=w301) -> ()  [unwired: 2 in, 2 out]
            n169 = property on="Test Slider" class="Slide (strict)"("Visible"=w301) -> ()  [unwired: 2 in, 2 out]
            n170 = property on="Test Ring" class="Ring (strict)"("Visible"=w301) -> ()  [unwired: 2 in, 2 out]
            n171 = property on="On/Off" class="Bool (strict)"("Visible"=TRUE, "Caption.Text"=w302) -> ()  [unwired: 2 in, 2 out]
            n172 = property on="Rev/Fwd" class="Clust (strict)"("Visible"=FALSE) -> ()  [unwired: 2 in, 2 out]
          }
          frame "Camera" {
            n173 = call <vilib>:"Get Last Path Segment.vi"("String in"=w309) -> ("String out"=w310:string)  [unwired: 10 in]
            n174 = property on="On/Off" class="Bool (strict)"("Visible"=FALSE) -> ()  [unwired: 2 in, 2 out]
            n175 = property on="Motor" class="Clust (strict)"("Visible"=FALSE) -> ()  [unwired: 2 in, 2 out]
            n176 = property on="Rev/Fwd" class="Clust (strict)"("Visible"=FALSE) -> ()  [unwired: 2 in, 2 out]
            n177 = case shown="\"White Balance  **\"" w310 {
              tunnel: w309 -> [w316 w325 w334 w343 w352 _ w358]
              tunnel: w308 -> [w314 w322 w331 w340 w349 _ _]
              frame "Size  **" {
                n178 = Index Array(array=w314) -> (element=w313:cluster{string[]})  [unwired: 1 in]
                n179 = call <vilib>:"NT Read String.vi"("Name"=w316) -> ("String"=w315:string)  [unwired: 9 in, 1 out]
                n180 = Unbundle(w313) -> (w311:string[])
                n181 = Match First String(2:w311, 3:w315) -> (0:w312:i32)  [unwired: 1 out]
                n182 = property on="Test Ring" class="Ring (strict)"("Value"=w312, "Strings []"=w311) -> ()  [unwired: 2 in, 2 out]
                n183 = property on="Test Ring" class="Ring (strict)"("Visible"=TRUE) -> ()  [unwired: 2 in, 2 out]
                n184 = property on="Test Slider" class="Slide (strict)"("Visible"=FALSE) -> ()  [unwired: 2 in, 2 out]
              }
              frame "White Balance  **" {
                n185 = Index Array(array=w322, index=1) -> (element=w323:cluster{string[]})
                n186 = call <vilib>:"NT Read String.vi"("Name"=w325) -> ("String"=w324:string)  [unwired: 9 in, 1 out]
                n187 = Unbundle(w323) -> (w320:string[])
                n188 = Match First String(2:w320, 3:w324) -> (0:w319:i32)  [unwired: 1 out]
                n189 = property on="Test Ring" class="Ring (strict)"("Value"=w319, "Strings []"=w320) -> ()  [unwired: 2 in, 2 out]
                n190 = property on="Test Ring" class="Ring (strict)"("Visible"=TRUE) -> ()  [unwired: 2 in, 2 out]
                n191 = property on="Test Slider" class="Slide (strict)"("Visible"=FALSE) -> ()  [unwired: 2 in, 2 out]
              }
              frame "Exposure  **" {
                n192 = Index Array(array=w331, index=2) -> (element=w332:cluster{string[]})
                n193 = call <vilib>:"NT Read String.vi"("Name"=w334) -> ("String"=w333:string)  [unwired: 9 in, 1 out]
                n194 = Unbundle(w332) -> (w328:string[])
                n195 = Match First String(2:w328, 3:w333) -> (0:w329:i32)  [unwired: 1 out]
                n196 = property on="Test Ring" class="Ring (strict)"("Value"=w329, "Strings []"=w328) -> ()  [unwired: 2 in, 2 out]
                n197 = property on="Test Ring" class="Ring (strict)"("Visible"=TRUE) -> ()  [unwired: 2 in, 2 out]
                n198 = property on="Test Slider" class="Slide (strict)"("Visible"=FALSE) -> ()  [unwired: 2 in, 2 out]
              }
              frame "Exposure Priority  **" {
                n199 = Index Array(array=w340, index=3) -> (element=w341:cluster{string[]})
                n200 = call <vilib>:"NT Read String.vi"("Name"=w343) -> ("String"=w342:string)  [unwired: 9 in, 1 out]
                n201 = Unbundle(w341) -> (w337:string[])
                n202 = Match First String(2:w337, 3:w342) -> (0:w338:i32)  [unwired: 1 out]
                n203 = property on="Test Ring" class="Ring (strict)"("Value"=w338, "Strings []"=w337) -> ()  [unwired: 2 in, 2 out]
                n204 = property on="Test Ring" class="Ring (strict)"("Visible"=TRUE) -> ()  [unwired: 2 in, 2 out]
                n205 = property on="Test Slider" class="Slide (strict)"("Visible"=FALSE) -> ()  [unwired: 2 in, 2 out]
              }
              frame "Color Enable  **" {
                n206 = Index Array(array=w349, index=4) -> (element=w350:cluster{string[]})
                n207 = call <vilib>:"NT Read String.vi"("Name"=w352) -> ("String"=w351:string)  [unwired: 9 in, 1 out]
                n208 = Unbundle(w350) -> (w346:string[])
                n209 = Match First String(2:w346, 3:w351) -> (0:w347:i32)  [unwired: 1 out]
                n210 = property on="Test Ring" class="Ring (strict)"("Value"=w347, "Strings []"=w346) -> ()  [unwired: 2 in, 2 out]
                n211 = property on="Test Ring" class="Ring (strict)"("Visible"=TRUE) -> ()  [unwired: 2 in, 2 out]
                n212 = property on="Test Slider" class="Slide (strict)"("Visible"=FALSE) -> ()  [unwired: 2 in, 2 out]
              }
              frame Default {
                n213 = property on="Test Ring" class="Ring (strict)"("Visible"=FALSE) -> ()  [unwired: 2 in, 2 out]
                n214 = property on="Test Slider" class="Slide (strict)"("Visible"=FALSE) -> ()  [unwired: 2 in, 2 out]
              }
              frame "Brightness  **", "Color Level  **", "Compression  **", "FPS  **", "Sharpness  **" {
                n215 = call <vilib>:"NT Read Number.vi"("Name"=w358) -> ("Numeric"=w357:dbl)  [unwired: 9 in, 1 out]
                n216 = local write "Test Slider"(w357) -> ()
                n217 = property on="Test Slider" class="Slide (strict)"("Visible"=TRUE, "Scale.Maximum"=100.0 ("Scale.Range:Maximum")) -> ()  [unwired: 2 in, 2 out]
                n218 = property on="Test Ring" class="Ring (strict)"("Visible"=FALSE) -> ()  [unwired: 2 in, 2 out]
              }
            }
          }
        }
        n219 = property on="Progress" class="Clust (strict)"("Visible"=FALSE) -> ()  [unwired: 2 in, 2 out]
      }
      event "Test Name": Mouse Enter {
        # "Populate the ring with the list of tests"
        n220 = event-data() -> ()  [unwired: 1 in, 1 out]
        n221 = call <vilib>:"NT Read String Array.vi"("Name"="TestMode/TestList") -> ("String Array"=w366:string[])  [unwired: 9 in, 1 out]
        n222 = Build Array (concatenate)("Select the test to run...", w366) -> (w365:string[])
        n223 = property on="Test Name" class="Ring (strict)"("Strings []"=w365) -> ()  [unwired: 2 in, 2 out]
      }
      event "Test Name": Value Change {
        w368 = FALSE ("Visible")
        # "Tell the robot the test name to run"
        n224 = event-data() -> ("NewVal"=w372:u16)  [unwired: 1 in]
        n225 = property on="Test Name" class="Ring (strict)"() -> ("Strings []"=w373:string[])  [unwired: 2 in, 2 out]
        n226 = local write "Progress"(T6 {"Test Progress"=0, "Test Progress Text"=""} ("Progress")) -> ()
        n227 = Index Array(array=w373, index=w372) -> (element=w371:string)
        n228 = call <vilib>:"NT Write String.vi"("String"=w371, "Name"="TestMode/TestName") -> ()  [unwired: 9 in, 1 out]
        n229 = property on="Progress" class="Clust (strict)"("Visible"=TRUE) -> ()  [unwired: 2 in, 2 out]
        n230 = property on="Motor" class="Clust (strict)"("Visible"=w368) -> ()  [unwired: 2 in, 2 out]
        n231 = property on="Test Slider" class="Slide (strict)"("Visible"=w368) -> ()  [unwired: 2 in, 2 out]
        n232 = property on="On/Off" class="Bool (strict)"("Visible"=w368) -> ()  [unwired: 2 in, 2 out]
        n233 = property on="Rev/Fwd" class="Clust (strict)"("Visible"=w368) -> ()  [unwired: 2 in, 2 out]
        n234 = property on="Test Ring" class="Ring (strict)"("Visible"=w368) -> ()  [unwired: 2 in, 2 out]
      }
      event "Select Auto": Mouse Enter {
        # "Populate the combo box with the list of autonomous options"
        n235 = event-data() -> ()  [unwired: 1 in, 1 out]
        n236 = call <vilib>:"NT Read String Array.vi"("Name"="Auto List") -> ("String Array"=w375:string[])  [unwired: 9 in, 1 out]
        n237 = property on="Select Auto" class="CmbBox"("Strings[]"=w375) -> ()  [unwired: 2 in, 2 out]
      }
      event "Select Auto": Value Change {
        # "User modified the Auto Selection. Write to NT variable so robot knows."
        n238 = event-data() -> ("NewVal"=w378:string)  [unwired: 1 in]
        n239 = call <vilib>:"NT Write String.vi"("String"=w378, "Name"="Auto Selector") -> ()  [unwired: 9 in, 1 out]
      }
      event "Command Selection": Value Change {
        # "Get the params and show in table"
        n240 = event-data() -> ("NewVal"=w384:i32)  [unwired: 1 in]
        n241 = property on="Command Selection" class="MCListbox (strict)"() -> ("ItemNames"=w382:string[][])  [unwired: 2 in, 2 out]
        n242 = call <vilib>:"WPI_DashboardUpdate Command Params.vi"("NewVal"=w384, "Commands"=w382, "Param Tbl"=w383) -> ()  [unwired: 8 in, 1 out]
      }
      event "Execute Command": Value Change {
        # "Started one, Unique ID holds\nresponse"
        n243 = event-data() -> ()  [unwired: 1 in, 1 out]
        n244 = property on="Command Selection" class="MCListbox (strict)"() -> ("ItemNames"=w395:string[][])  [unwired: 2 in, 2 out]
        n245 = Index Array(array=w395, index (row)="Command Selection", index (col)=0) -> (element=w393:string)
        n246 = call <vilib>:"Invoke Commands.vi"("Command Params"="Command Params", "Function Name"=w393) -> ("Params"=w389:u8, "Started"=w388:bool)  [unwired: 7 in, 1 out]
        n247 = Array Subset(array="Command Params", length (row)=w389) -> (w390:string[][])  [unwired: 3 in]
        n248 = Select(t="Executing" ("Cmd Status"), s=w388, f="" ("Cmd Status")) -> (s? t:f=→"Cmd Status":string)
      }
      event "Command Selection": Double Click {
        n249 = event-data() -> ("Row"=w403:i32)  [unwired: 1 in]
        n250 = property on="Command Selection" class="MCListbox (strict)"() -> ("ItemNames"=w406:string[][])  [unwired: 2 in, 2 out]
        n251 = local read "Command Params"() -> (w402:string[][])
        n252 = Index Array(array=w406, index (row)=w403, index (col)=0) -> (element=w404:string)
        n253 = call <vilib>:"Invoke Commands.vi"("Command Params"=w402, "Function Name"=w404) -> ("Params"=w401:u8, "Started"=w396:bool)  [unwired: 7 in, 1 out]
        n254 = Array Subset(array=w402, length (row)=w401) -> (w400:string[][])  [unwired: 3 in]
        n255 = Select(t="Executing" ("Cmd Status"), s=w396, f="" ("Cmd Status")) -> (s? t:f=w397:string)
        n256 = local write "Cmd Status"(w397) -> ()
      }
      event "CheckList": Double Click {
        # "Shift clears all"
        # "Update symbols on the listbox"
        n257 = event-data() -> ("PlatMods.Shift"=w408:bool, "Row"=w410:i32)  [unwired: 1 in]
        n258 = case shown="True" w408 {
          tunnel: w410 -> [w414 _]
          tunnel: 1 -> [w413 _]
          frame False {
            n259 = property on="CheckList" class="LstBox (strict)"() -> ("Item Symbols"=w412:i32[])  [unwired: 2 in, 2 out]
            n260 = Replace Array Subset(array=w412, new element=w413, index=w414) -> (w411:i32[])
            n261 = property on="CheckList" class="LstBox (strict)"("Item Symbols"=w411) -> ()  [unwired: 2 in, 2 out]
          }
          frame True {
            w415 = 0 ("Top Row")
            n262 = property on="CheckList" class="LstBox (strict)"() -> ("Number of Rows"=w417:u32)  [unwired: 2 in, 2 out]
            n263 = Initialize Array(0, w417) -> (w416:i32[])
            n264 = property on="CheckList" class="LstBox (strict)"("Top Row"=w415, "Value"=w415, "Item Symbols"=w416) -> ()  [unwired: 2 in, 2 out]
          }
        }
      }
      event "CheckList": Key Down {
        # "Update symbols on the listbox\nLeft and right keys check and uncheck"
        n265 = event-data() -> ("VKey"=w421:T27)  [unwired: 1 in]
        n266 = case shown="\"Left\", \"Right\"" w421 {
          selector: w421 -> [w426 _]
          tunnel: eventvkey."Left" ("VKey") -> [w424 _]
          frame "Left", "Right" {
            n267 = Equal?(x=w424, y=w426) -> (x = y?=w425:bool)
            n268 = Select(t=0, s=w425, f=1) -> (s? t:f=w427:i32)
            n269 = property on="CheckList" class="LstBox (strict)"() -> ("Item Symbols"=w430:i32[])  [unwired: 2 in, 2 out]
            n270 = Replace Array Subset(array=w430, new element=w427, index="CheckList") -> (w429:i32[])
            n271 = property on="CheckList" class="LstBox (strict)"("Item Symbols"=w429) -> ()  [unwired: 2 in, 2 out]
          }
          frame Default {
          }
        }
      }
      event "Motor.Enable": Value Change {
        # "When the test mode otor enable helper is set, update that\ntree row item's value"
        n272 = event-data() -> ("NewVal"=w436:bool)  [unwired: 1 in]
        n273 = Unbundle("Motor") -> ("Value"=w435:dbl)  [unwired: 1 out]
        n274 = Select(t=w435, s=w436, f=0.0) -> (s? t:f=w433:dbl)
        n275 = call <vilib>:"NT Write Number.vi"("Numeric"=w433, "Name"=w432) -> ()  [unwired: 9 in, 1 out]
      }
      event "Test Slider": Value Change {
        # "When the test mode slider helper is set, update that\ntree row item's value"
        n276 = event-data() -> ("NewVal"=w439:dbl)  [unwired: 1 in]
        n277 = call <vilib>:"NT Write Number.vi"("Numeric"=w439, "Name"=w440) -> ()  [unwired: 9 in, 1 out]
      }
      event "On/Off": Value Change {
        # "When the test mode on/off helper value is set, update that\ntree row item's value"
        n278 = event-data() -> ("NewVal"=w444:bool)  [unwired: 1 in]
        n279 = Boolean To (0,1)(Boolean=w444) -> (0, 1=w443:i16)
        n280 = call <vilib>:"NT Write Number.vi"("Numeric"=w443, "Name"=w442) -> ()  [unwired: 9 in, 1 out]
      }
      event "Rev/Fwd": Value Change {
        # "When the test mode helper value for relays is set, update that\ntree row item's value"
        n281 = event-data() -> ("NewVal.Forward"=w452:bool, "NewVal.Reverse"=w451:bool)  [unwired: 1 in]
        n282 = Boolean To (0,1)(Boolean=w452) -> (0, 1=w448:i16)
        n283 = Boolean To (0,1)(Boolean=w451) -> (0, 1=w450:i16)
        n284 = Negate(x=w450) -> (-x=w449:i16)
        n285 = Add(x=w448, y=w449) -> (x+y=w447:i16)
        n286 = call <vilib>:"NT Write Number.vi"("Numeric"=w447, "Name"=w446) -> ()  [unwired: 9 in, 1 out]
      }
      event "Test Ring": Value Change {
        # "When a test mode helper value is selected from the ring,\nset the tree item's variable to the string value"
        n287 = event-data() -> ("NewVal"=w456:u16)  [unwired: 1 in]
        n288 = property on="Test Ring" class="Ring (strict)"() -> ("Strings []"=w457:string[])  [unwired: 2 in, 2 out]
        n289 = Index Array(array=w457, index=w456) -> (element=w455:string)
        n290 = call <vilib>:"NT Write String.vi"("String"=w455, "Name"=w454) -> ()  [unwired: 9 in, 1 out]
      }
      event "Rec Mode": Value Change {
        # "Update globals for recording mode and path to read log from.\nClear when logging and let NetworkTables set path for vision to\nuse."
        n291 = event-data() -> ("NewVal"=w468:enum32{"Stop", "Record", "Playback"})  [unwired: 1 in]
        n292 = global write "WPI_DashboardLogging Global.vi" "Logging Filename"(path "") -> ()
        n293 = global write "WPI_DashboardLogging Global.vi" "Recording"(w468) -> ()
        n294 = case shown="\"Playback\"" w468 {
          tunnel: w467 -> [_ w470 w479]
          tunnel: [_ _ w478] -> w465
          tunnel: [_ _ w477] -> _
          tunnel: w463 -> [_ _ w475]
          tunnel: cluster{i32, i32} {-250, 170} -> [_ _ w474]
          tunnel: [_ _ T28 {"Image Size"=TRUE, "Image Type"=TRUE, "Pixel Value"=TRUE, "ROI Information"=TRUE, "Zoom Factor"=FALSE} ("Image Information Shown:All Elements")] -> w458
          tunnel: [_ _ TRUE ("Zoom Factor")] -> w459
          tunnel: w461 -> [_ _ w471]
          frame Default {
          }
          frame "Stop", "Record" {
            # "Place Window too"
            n295 = invoke class="VI" method="FP.Close"(reference=w470) -> (reference out=w469:refnum<vi>)  [unwired: 2 in, 2 out]
            n296 = invoke class="VI" method="Abort VI"(reference=w469) -> ()  [unwired: 2 in, 3 out]
          }
          frame "Playback" {
            n297 = call "Open Playback Panel.vi"("Offset"=w474, "DB VI Ref"=w475, "Playback in"=w479) -> ("Playback out"=w476:refnum<vi>)  [unwired: 8 in]
            n298 = register-events(w476, w471) -> (reference out=w478:refnum<event-registration>, error out=w477:errorcluster)  [unwired: 2 in]
          }
        }
        n299 = property on="Camera Image Right" class="ImageControl"("Image Information Shown"=w458, "Image Information Visible"=w459) -> ()  [unwired: 2 in, 2 out]
        n300 = property on="Camera Image" class="ImageControl"("Image Information Shown"=w458, "Image Information Visible"=w459) -> ()  [unwired: 2 in, 2 out]
        n301 = call <vilib>:"WPI_DashboardNT Log FieldName Cache.vi"("Operation"=enum16{"Lookup/Add", "Index", "Clear"}."Clear") -> ()  [unwired: 8 in, 3 out]
      }
      event Panel Close {
        w481 = enum32{"Stop", "Record", "Playback"}."Stop" ("Rec Mode")
        # "Playback window has been closed, abort"
        n302 = event-data() -> ()  [unwired: 1 in, 4 out]
        n303 = local write "Rec Mode"(w481) -> ()
        n304 = global write "WPI_DashboardLogging Global.vi" "Recording"(w481) -> ()
      }
      event Panel Close {
        # "Abort playback window and ourself"
        n305 = event-data() -> ()  [unwired: 1 in, 4 out]
        n306 = invoke class="VI" method="FP.Close"(reference=w485) -> (reference out=w484:refnum<vi>)  [unwired: 2 in, 2 out]
        n307 = invoke class="VI" method="Abort VI"(reference=w484) -> (error out=w483:errorcluster)  [unwired: 2 in, 2 out]
        n308 = invoke class="VI" method="Abort VI"(error in=w483) -> ()  [unwired: 2 in, 3 out]
      }
      event User Event {
        n309 = event-data() -> ("IDs"=w492:cluster{"RPC field ID":u16, "Unique ID":u16}, "String"=w491:string)  [unwired: 1 in]
        n310 = Bundle("IDs"=w492, "String"=w491) -> (w490:T9)  [unwired: 1 in]
        n311 = call <vilib>:"Retrieve RPC Response.vi"("RPC Response"=w490) -> ("Output"=w488:string[][])  [unwired: 10 in]
        n312 = Build Array (concatenate)(w486, w488) -> (w487:string[][])
        n313 = local write "Command Params"(w487) -> ()
        n314 = local write "Cmd Status"("" ("Cmd Status")) -> ()
      }
      event "Tree": Double Click {
        n315 = event-data() -> ("PlatMods"=w498:T31, "Tag"=w495:string)  [unwired: 1 in]
        n316 = Unbundle(w498) -> ("Shift"=w497:bool)  [unwired: 4 out]
        n317 = String Subset(string=w495, length (rest)=1 ("length (rest)")) -> (substring=w494:string)  [unwired: 1 in]
        n318 = Not(x=w497) -> (.not. x?=w496:bool)
        n319 = case shown="\"/\"" w494 {
          tunnel: w495 -> [_ w501]
          tunnel: w496 -> [_ w500]
          frame Default {
          }
          frame "/" {
            n320 = call <vilib>:"NT Update Persistence.vi"("Persistence"=w500, "Name"=w501) -> ()  [unwired: 9 in, 1 out]
          }
        }
      }
    }
  }
  n321 = while {
    tunnel: w70 -> [w503]
    i -> [w506]
    stop <- FALSE stop-if-true
    n322 = Wait (ms)(milliseconds to wait=u32 100) -> ()  [unwired: 1 out]
    n323 = case shown="\"Playback\"" "Rec Mode" {
      tunnel: w506 -> [_ _ w521]
      tunnel: [u32 2829099 ("Base Color") u32 11141120 ("Target Color") w510] -> w502
      frame "Stop", Default {
        # "Reset the color, extra updates don't cost much"
      }
      frame "Record" {
      }
      frame "Playback" {
        # "Playback"
        n324 = Quotient & Remainder(x=w521, y=u32 50 ("milliseconds to wait")) -> (x-y*floor(x/y)=w517:u32)  [unwired: 1 out]
        n325 = Divide(x=w517, y=u32 50 ("milliseconds to wait")) -> (x/y=w514:dbl)
        n326 = Multiply(x=6.283185307179586, y=w514) -> (x*y=w519:dbl)
        n327 = Sine(x=w519) -> (sin(x)=w518:dbl)
        n328 = Absolute Value(x=w518) -> (abs(x)=w511:dbl)
        n329 = call "Interpolate RGB Color.vi"("Proportion"=w511, "Target Color"=u32 30976, "Base Color"=u32 2829099) -> ("Result Color"=w510:u32)  [unwired: 8 in]
      }
    }
    n330 = property class="Pane"(reference=w503, "PaneColor"=w502) -> ()  [unwired: 1 in, 2 out]
  }
  n331 = local write "Dashboard Tab"(T2."Drive" ("Dashboard Tab")) -> ()
  n332 = property on="On/Off" class="Bool (strict)"("Visible"=w41) -> ()  [unwired: 2 in, 2 out]
  n333 = property on="Motor" class="Clust (strict)"("Visible"=w41) -> ()  [unwired: 2 in, 2 out]
  n334 = property on="Progress" class="Clust (strict)"("Visible"=w41) -> ()  [unwired: 2 in, 2 out]
  n335 = property on="Test Ring" class="Ring (strict)"("Visible"=w41) -> ()  [unwired: 2 in, 2 out]
  n336 = property on="Rev/Fwd" class="Clust (strict)"("Visible"=w41) -> ()  [unwired: 2 in, 2 out]
  n337 = while {
    tunnel: u16 1741 ("timeout ms (25000)") -> [w523]
    stop <- FALSE stop-if-true
    n338 = TCP Create Listener(10:w523) -> (0:w522:errorcluster, 3:w524:refnum<k5>)  [unwired: 4 in, 1 out]
    n339 = case shown="No Error" w522 {
      selector: w522 -> [w526 _]
      tunnel: w524 -> [w527 _]
      frame No Error {
        n340 = while {
          tunnel: w527 -> [w530]
          tunnel: w526 -> [w529]
          stop <- FALSE stop-if-true
          n341 = TCP Wait On Listener(8:w529, 11:w530) -> (0:w531:errorcluster, 4:w532:refnum<k5>)  [unwired: 2 in, 3 out]
          n342 = local write "TCP"(w532) -> ()
          n343 = case shown="No Error" w531 {
            frame No Error {
            }
            frame Error {
              n344 = Wait (ms)(milliseconds to wait=u32 1000) -> ()  [unwired: 1 out]
            }
          }
        }
      }
      frame Error {
        n345 = Wait (ms)(milliseconds to wait=u32 1000) -> ()  [unwired: 1 out]
      }
    }
  }
  n346 = local write "Command Selection"(u16 0 ("milliseconds to wait")) -> ()
  n347 = local write "Command Params"(string[][] [] ("Command Params")) -> ()
  n348 = global write "WPI_DashboardLogging Global.vi" "Recording"(w64) -> ()
  n349 = local write "Rec Mode"(w64) -> ()
  n350 = call <vilib>:"NT Write String.vi"("String"="Select Auto", "Name"="Auto Selector") -> ()  [unwired: 9 in, 1 out]
  n351 = call <vilib>:"Close.vi"("Error In"=w1, "LINX Resource"=w2) -> ()  [unwired: 9 in, 1 out]
